vi "GetInfo.vi"(11 "File selected":T2) -> (2 "remove?":bool)   [LabVIEW 2022 SP3]
uses:
  Curtin1_Label.ctl
panel:
  in  "Instruments":u16(ring) items=["ME45 01 H.AvR", "ME45 02 H.AvR", "ME45 03 H.AvR"]
  in  "Play":bool
  in  "View Raw Data":bool
  in  "Open":bool
  out "Block":bool
  in  "Done 2":bool
  out "Instrument--Test":string
  in  "Recalc":bool
  in  "Overwrite":bool
  in  "Settings":T1={"Name of test"="", "Date"=timestamp(0 s since 1904-01-01), "Location"="", "Default Template"="", "Soundcard"="", "resolution"=32, "Sampling rate"=48000, "Ch1 Gain "=25.0, "Ch2 Gain"=10.0, "Sample time (s)"=0.3, "Pre-trigger (s)"=0.01, "Hammer Threshold"=10.0, "Positions"=12, "Taps/Position"=5, "Set Names"="", "Freq resolution"=10.0, "Hammer cutoff"=0.0, "Mic cutoff"=0.0, "Double bounce "=0.0, "Hammer Cal"=10.0, "dB Offset"=0.0, "Accel Cal"=10.0, "Vibrometer Cal"=0.0, "Mic Cal"=0.0, "Output"=2, "Voltage Cal"=0.01, "Vibrometer Port"="ASRL27::INSTR", "Range"=4, "High Pass"=2, "Bandwidth"=4, "X Range"=[{"Minimum"=200.0, "Maximum"=10000.0, "Increment"=10.0, "Minor Increment"=100.0, "Start"=200.0}, {"Minimum"=0.0, "Maximum"=0.05, "Increment"=0.025, "Minor Increment"=0.0025, "Start"=0.0}, {"Minimum"=0.0, "Maximum"=0.3, "Increment"=0.1, "Minor Increment"=0.01, "Start"=0.0}, {"Minimum"=200.0, "Maximum"=10000.0, "Increment"=10.0, "Minor Increment"=100.0, "Start"=1000.0}], "Y Range"=[{"Minimum"=-25.0, "Maximum"=0.0, "Increment"=5.0, "Minor Increment"=1.0, "Start"=-25.0}, {"Minimum"=-0.01, "Maximum"=0.1, "Increment"=0.02, "Minor Increment"=0.005, "Start"=0.0}, {"Minimum"=-0.1, "Maximum"=0.1, "Increment"=0.05, "Minor Increment"=0.01, "Start"=-0.1}, {"Minimum"=-35.0, "Maximum"=5.0, "Increment"=2.0, "Minor Increment"=0.5, "Start"=-34.0}], "dB Spread"=0.0, "Trigger"=0, "Ch_1"=25, "Ch_2"=25, "flip?"=FALSE, "60Hz"=FALSE, "Time offset"=0.0, "Piezo Cal"=0.0, "Default Notes"=""} {"Ch_2" min=1 step=1; "Ch_1" min=1 max=100 step=1; "Trigger" items=["Hammer (force)", "Self-tap"]; "Bandwidth" items=["1 kHz", "5 kHz", "10 kHz", "25 kHz", "50 kHz", "100 kHz"]; "High Pass" items=["Off", "13 Hz", "104 Hz"]; "Range" items=["10 mm/s", "20 mm/s", "50 mm/s", "100 mm/s", "200 mm/s", "500 mm/s", "1 m/s", "2 m/s"]; "Output" items=["Acclerometer", "Displacement", "Microphone", "Vibrometer"]; "Voltage Cal" format="%#_13g"; "Ch2 Gain" format="%#_13g"; "Ch1 Gain" format="%#_13g"; "Hammer Cal" min=0.0; "Double bounce" min=0.0; "Mic cutoff" min=0.0 format="%#_4g"; "Hammer cutoff" min=0.0 format="%#_4g"; "Freq resolution" min=0.0; "Pre-trigger (s)" format="%#_13g"; "Date" format="%<%H:%M\n%d/%m/%y>T"; "resolution" items=["16 bit"=16, "24 bit"=24, "32 bit"=32]; "Sampling rate" items=["22050 samp/s"=22050, "44100 samp/s"=44100, "48000 samp/s"=48000]}
  in  "Save as a Template":bool
  in  "Save":bool
  in  "Done":bool
  out "Tags":string
  in  "Notes":string
  out "File name":string
  # "mV/Pa"
  # "mV/m/s2"
  # "mV/mm/s"
  # "V/N"
  # "sec"
  # "sec"
  # "mV/N"
  # "Hz"
  # "a.u."
  # "dB"
  # "a.u."
  # "dB"
  # "sec"
  # "sec"
  # "sec"
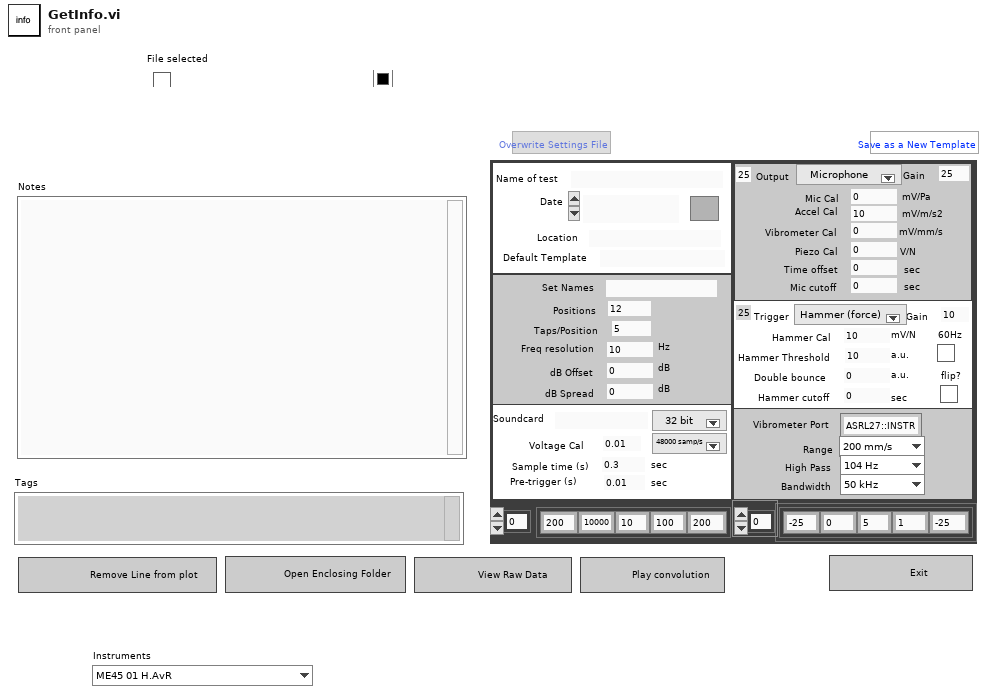
[diagram p1: front panel]
types:
  T1 = cluster{"Name of test":string, "Date":timestamp, "Location":string, "Default Template":string, "Soundcard":string, "resolution":u16, "Sampling rate":u16, "Ch1 Gain ":dbl, "Ch2 Gain":dbl, "Sample time (s)":dbl, "Pre-trigger (s)":dbl, "Hammer Threshold":dbl, "Positions":i16, "Taps/Position":i16, "Set Names":string, "Freq resolution":dbl, "Hammer cutoff":dbl, "Mic cutoff":dbl, "Double bounce ":dbl, "Hammer Cal":dbl, "dB Offset":dbl, "Accel Cal":dbl, "Vibrometer Cal":dbl, "Mic Cal":dbl, "Output":u16, "Voltage Cal":dbl, "Vibrometer Port":string, "Range":u16, "High Pass":u16, "Bandwidth":u16, "X Range":cluster{"Minimum":dbl, "Maximum":dbl, "Increment":dbl, "Minor Increment":dbl, "Start":dbl}[], "Y Range":cluster{"Minimum":dbl, "Maximum":dbl, "Increment":dbl, "Minor Increment":dbl, "Start":dbl}[], "dB Spread":dbl, "Trigger":u16, "Ch_1":u8, "Ch_2":u8, "flip?":bool, "60Hz":bool, "Time offset":dbl, "Piezo Cal":dbl, "Default Notes":string}
  T2 = typedef "Curtin1_Label.ctl" = cluster{"Show?":bool, "Name":string, "Color":u32, "Path":path, "Show Notes":bool}
  T3 = enum8{"Enabled", "Disabled", "Disabled and Grayed Out"}
  T4 = cluster{"Name of test":string, "Date":timestamp, "Location":string, "Template":string, "Soundcard":string, "resolution":u16, "Sampling rate":u16, "Ch1 Gain ":dbl, "Ch2 Gain":dbl, "Sample time (s)":dbl, "Pre-trigger (s)":dbl, "Hammer Threshold":dbl, "Positions":i16, "Taps/Position":i16, "Set Names":string, "Freq resolution":dbl, "Hammer cutoff":dbl, "Mic cutoff":dbl, "Double bounce ":dbl, "Hammer Cal":dbl, "dB Offset":dbl, "Accel Cal":dbl, "Vibrometer Cal":dbl, "Mic Cal":dbl, "Output":u16, "Voltage Cal":dbl, "Vibrometer Port":string, "Range":u16, "High Pass":u16, "Bandwidth":u16, "X Range":cluster{"Minimum":dbl, "Maximum":dbl, "Increment":dbl, "Minor Increment":dbl, "Start":dbl}[], "Y Range":cluster{"Minimum":dbl, "Maximum":dbl, "Increment":dbl, "Minor Increment":dbl, "Start":dbl}[], "dB Spread":dbl, "Trigger":u16, "Ch_1":u8, "Ch_2":u8, "flip?":bool, "60Hz":bool, "Time offset":dbl, "Piezo Cal":dbl, "Default Notes":string}
  T5 = enum32{"Invalid", "Default", "Floating", "Floating/Auto-Hide", "Modal"}
  T6 = typedef "PreferencesControl.ctl" = cluster{"Name of test":string, "Date":timestamp, "Location":string, "Template":string, "Soundcard":string, "resolution":u16, "Sampling rate":u16, "Ch1 Gain ":dbl, "Ch2 Gain":dbl, "Sample time (s)":dbl, "Pre-trigger (s)":dbl, "Hammer Threshold":dbl, "Positions":i16, "Taps/Position":i16, "Set Names":string, "Freq resolution":dbl, "Hammer cutoff":dbl, "Mic cutoff":dbl, "Double bounce ":dbl, "Hammer Cal":dbl, "dB Offset":dbl, "Accel Cal":dbl, "Vibrometer Cal":dbl, "Mic Cal":dbl, "Output":u16, "Voltage Cal":dbl, "Vibrometer Port":refnum<visa-resource-name>, "Range":u16, "High Pass":u16, "Bandwidth":u16, "X Range":cluster{"Minimum":dbl, "Maximum":dbl, "Increment":dbl, "Minor Increment":dbl, "Start":dbl}[], "Y Range":cluster{"Minimum":dbl, "Maximum":dbl, "Increment":dbl, "Minor Increment":dbl, "Start":dbl}[], "dB Spread":dbl, "Trigger":u16, "Ch_1":u8, "Ch_2":u8, "flip?":bool, "60Hz":bool, "Time offset":dbl, "Piezo Cal":dbl, "Default Notes":string}
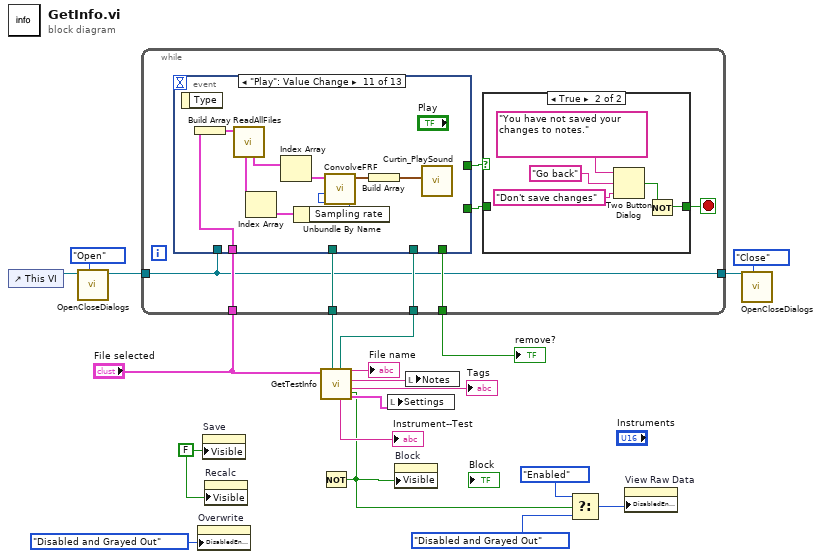
[diagram p0: block diagram]
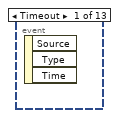
[diagram p3: hidden frame]
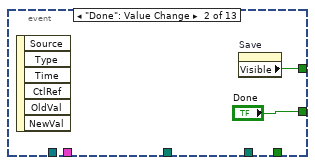
[diagram p4: hidden frame]
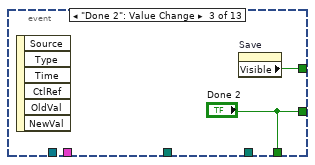
[diagram p5: hidden frame]
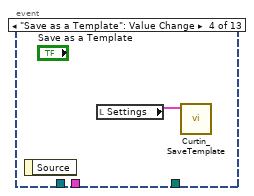
[diagram p6: hidden frame]
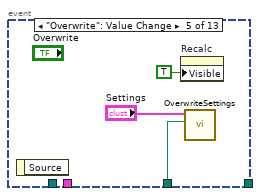
[diagram p7: hidden frame]
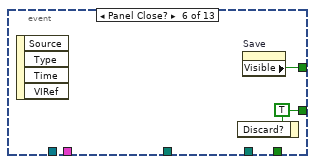
[diagram p8: hidden frame]
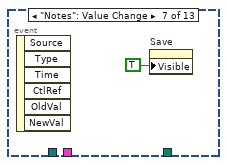
[diagram p9: hidden frame]
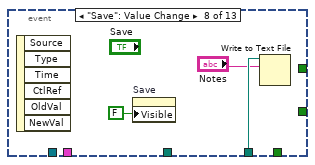
[diagram p10: hidden frame]
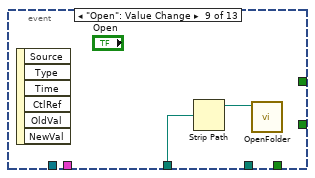
[diagram p11: hidden frame]
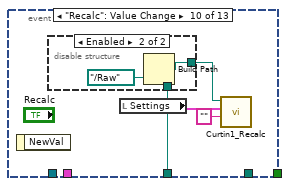
[diagram p12: hidden frame]
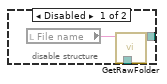
[diagram p13: hidden frame]
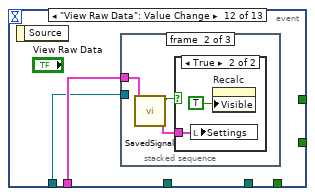
[diagram p14: hidden frame]
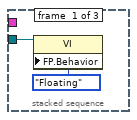
[diagram p15: hidden frame]
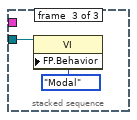
[diagram p17: hidden frame]
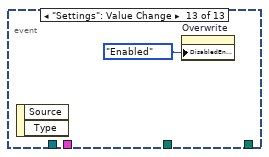
[diagram p18: hidden frame]
diagram:
  w21 = FALSE ("Visible")
  n1 = control-ref of="This VI"() -> (w10:refnum<vi>)
  n2 = call "OpenCloseDialogs.vi"("Task"=enum16{"Open", "Close"}."Open", "VI in"=w10) -> ("VI out"=w7:refnum<vi>)  [unwired: 8 in, 1 out]
  n3 = property on="Overwrite" class="Bool"("DisabledEnum"=T3."Disabled and Grayed Out" ("Disabled")) -> ()  [unwired: 2 in, 2 out]
  n4 = property on="Save" class="Bool"("Visible"=w21) -> ()  [unwired: 2 in, 2 out]
  n5 = property on="Recalc" class="Bool"("Visible"=w21) -> ()  [unwired: 2 in, 2 out]
  n6 = call "GetTestInfo.vi"("File selected"="File selected") -> ("Settings"=w16:T4, "Tags"=→"Tags":string, "Notes"=w18:string, "File name"=→"File name":string, "Instrument--Test"=→"Instrument--Test":string, "Notes Path"=w13:path, "Visible?"=w3:bool, "Settings Path"=w14:path)  [unwired: 3 in]
  n7 = while {
    tunnel: w13 -> [w29]
    tunnel: w14 -> [w25]
    tunnel: [w24] -> w12
    tunnel: [w22] -> w8
    tunnel: w7 -> [w22]
    tunnel: "File selected" -> [w23]
    stop <- w26 stop-if-true
    n8 = event shown="[10] \"Play\": Value Change" {
      selector: _ -> [_ _ _ _ _ _ _ _ _ _ _ _ _]
      dyn-events: _ -> [_ _ _ _ _ _ _ _ _ _ _ _ _]
      timeout: _ -> [_ _ _ _ _ _ _ _ _ _ _ _ _]
      tunnel: w29 -> [_ _ _ _ _ _ _ w49 _ _ _ _ _]
      tunnel: [_ w37 w39 _ _ w45 _ _ _ _ _ _ _] -> w28
      tunnel: [_ "Done" "Done 2" _ _ w44 _ _ _ _ _ _ _] -> w27
      tunnel: w25 -> [_ _ _ _ w42 _ _ _ w51 w52 _ _ _]
      tunnel: [_ _ "Done 2" _ _ _ _ _ _ _ _ _ _] -> w24
      tunnel: w23 -> [_ _ _ _ _ _ _ _ _ _ w62 w71 _]
      tunnel: w22 -> [_ _ _ _ _ _ _ _ _ _ _ w70 _]
      event Timeout {
        n9 = event-data() -> ()  [unwired: 1 in, 3 out]
      }
      event "Done": Value Change {
        n10 = event-data() -> ()  [unwired: 1 in, 6 out]
        n11 = property on="Save" class="Bool"() -> ("Visible"=w37:bool)  [unwired: 2 in, 2 out]
      }
      event "Done 2": Value Change {
        n12 = event-data() -> ()  [unwired: 1 in, 6 out]
        n13 = property on="Save" class="Bool"() -> ("Visible"=w39:bool)  [unwired: 2 in, 2 out]
      }
      event "Save as a Template": Value Change {
        n14 = event-data() -> ()  [unwired: 1 in, 1 out]
        n15 = local read "Settings"() -> (w40:T1)
        n16 = call "Curtin_SaveTemplate.vi"("Settings in"=w40) -> ()  [unwired: 8 in, 3 out]
      }
      event "Overwrite": Value Change {
        n17 = event-data() -> ()  [unwired: 1 in, 1 out]
        n18 = property on="Recalc" class="Bool"("Visible"=TRUE) -> ()  [unwired: 2 in, 2 out]
        n19 = call "OverwriteSettings.vi"("Settings path"=w42, "Settings"="Settings") -> ()  [unwired: 9 in, 1 out]
      }
      event Panel Close? {
        w44 = TRUE ("Done")
        n20 = event-data() -> ()  [unwired: 1 in, 4 out]
        n21 = event-data("Discard?"=w44) -> ()  [unwired: 1 in, 1 out]
        n22 = property on="Save" class="Bool"() -> ("Visible"=w45:bool)  [unwired: 2 in, 2 out]
      }
      event "Notes": Value Change {
        n23 = event-data() -> ()  [unwired: 1 in, 6 out]
        n24 = property on="Save" class="Bool"("Visible"=TRUE) -> ()  [unwired: 2 in, 2 out]
      }
      event "Save": Value Change {
        n25 = event-data() -> ()  [unwired: 1 in, 6 out]
        n26 = property on="Save" class="Bool"("Visible"=FALSE) -> ()  [unwired: 2 in, 2 out]
        n27 = Write to Text File(file (use dialog)=w49, text="Notes") -> ()  [unwired: 2 in, 3 out]
      }
      event "Open": Value Change {
        n28 = event-data() -> ()  [unwired: 1 in, 6 out]
        n29 = Strip Path(path=w51) -> (stripped path=w50:path)  [unwired: 1 out]
        n30 = call "OpenFolder.vi"("LabVIEW Data Path"=w50) -> ()  [unwired: 11 in]
      }
      event "Recalc": Value Change {
        n31 = event-data() -> ()  [unwired: 1 in, 1 out]
        n32 = disable-structure shown="Enabled" {
          disable-tunnel: [w56 w58] -> w53
          disable-tunnel: w52 -> [_ w59]
          frame Disabled {
            n33 = local read "File name"() -> (w57:string)
            n34 = call "GetRawFolder.vi"("File name"=w57) -> ("Path to Raw data"=w56:path)  [unwired: 10 in]
          }
          frame Enabled {
            n35 = Build Path(base path=w59, name or relative path=path "../Raw") -> (appended path=w58:path)
          }
        }
        n36 = local read "Settings"() -> (w55:T1)
        n37 = call "Curtin1_Recalc.vi"("Instrument:Test Name"="", "Settings"=w55, "Path To Raw Folder"=w53) -> ()  [unwired: 9 in]
      }
      event "Play": Value Change {
        n38 = event-data() -> ()  [unwired: 1 in, 1 out]
        n39 = Build Array(w62) -> (w61:T2[])
        n40 = call "ReadAllFiles.vi"("Files"=w61) -> ("data"=w63:cluster{"t0":dbl, "df":dbl, "Y":cdb[]}[], "Settings"=w65:T6[])  [unwired: 5 in, 4 out]
        n41 = Index Array(array=w65) -> (element=w66:T6)  [unwired: 1 in]
        n42 = Index Array(array=w63) -> (element=w64:cluster{"t0":dbl, "df":dbl, "Y":cdb[]})  [unwired: 1 in]
        n43 = Unbundle By Name(w66) -> ("Sampling rate"=w67:u16)
        n44 = call "ConvolveFRF.vi"("Sampling rate"=w67, "Complex FRF"=w64) -> ("Convolution"=w68:waveform(dbl))  [unwired: 7 in, 2 out]
        n45 = Build Array(w68) -> (w69:waveform(dbl)[])
        n46 = call "Curtin_PlaySound.vi"("all waveforms"=w69) -> ()  [unwired: 10 in, 1 out]
      }
      event "View Raw Data": Value Change {
        n47 = event-data() -> ()  [unwired: 1 in, 1 out]
        n48 = stacked-sequence {
          tunnel: w71 -> [_ w76 _]
          tunnel: w70 -> [w72 _ w79]
          frame #0 {
            n49 = property class="VI"(reference=w72, "FP.Behavior"=T5."Floating" ("Front Panel Window:Behavior")) -> ()  [unwired: 1 in, 2 out]
          }
          frame #1 {
            n50 = call "SavedSignal.vi"("File selected"=w76) -> ("Settings out"=w74:T6, "update?"=w75:bool)  [unwired: 9 in]
            n51 = case shown="True" w75 {
              tunnel: w74 -> [_ w77]
              frame False {
              }
              frame True {
                n52 = local write "Settings"(w77) -> ()
                n53 = property on="Recalc" class="Bool"("Visible"=TRUE) -> ()  [unwired: 2 in, 2 out]
              }
            }
          }
          frame #2 {
            n54 = property class="VI"(reference=w79, "FP.Behavior"=T5."Modal" ("Front Panel Window:Behavior")) -> ()  [unwired: 1 in, 2 out]
          }
        }
      }
      event "Settings": Value Change {
        n55 = event-data() -> ()  [unwired: 1 in, 2 out]
        n56 = property on="Overwrite" class="Bool"("DisabledEnum"=T3."Enabled" ("Disabled")) -> ()  [unwired: 2 in, 2 out]
      }
    }
    n57 = case shown="True" w28 {
      tunnel: [w30 w31] -> w26
      tunnel: w27 -> [w30 _]
      frame False {
      }
      frame True {
        n58 = Two Button Dialog(message="You have not saved your changes to notes.", 1:"Don't save changes" ("F button name (\"Cancel\")"), 2:"Go back" ("T button name (\"OK\")")) -> (T button?=w32:bool)
        n59 = Not(x=w32) -> (.not. x?=w31:bool)
      }
    }
  }
  "remove?" <- w12
  n60 = Not(x=w3) -> (.not. x?=w5:bool)
  n61 = local write "Settings"(w16) -> ()
  n62 = property on="Block" class="Bool (strict)"("Visible"=w5) -> ()  [unwired: 2 in, 2 out]
  n63 = local write "Notes"(w18) -> ()
  n64 = Select(t=T3."Enabled" ("Disabled"), s=w3, f=T3."Disabled and Grayed Out" ("Disabled")) -> (s? t:f=w1:T3)
  n65 = property on="View Raw Data" class="Bool"("DisabledEnum"=w1) -> ()  [unwired: 2 in, 2 out]
  n66 = call "OpenCloseDialogs.vi"("Task"=enum16{"Open", "Close"}."Close", "VI in"=w8) -> ()  [unwired: 8 in, 2 out]
